vi "Cache_Hierarchy Global_Write.vi"(10 "Class Hierarchies":T1[](array[typedef]), 11 "Class Names":string[](array[string])) -> (3 "Hierarchy Map":map{string, string[]}(c390))   [LabVIEW 2019, in "ClassLoader.lvlib"]
uses:
  ClassLoader.lvlib
  Cache_Hierarchy Global.vi
  Ctl/Ctl_Hierarchy Cluster.ctl
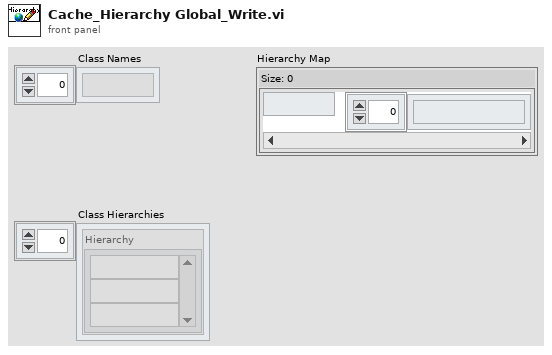
[diagram p1: front panel]
types:
  T1 = typedef "ClassLoader.lvlib/Ctl_Hierarchy Cluster.ctl" = cluster{"Hierarchy":string[]}
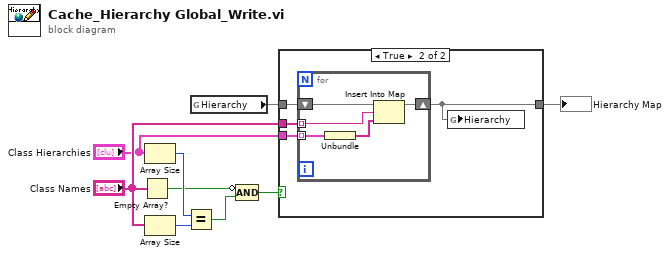
[diagram p0: block diagram]
diagram:
  n1 = Empty Array?(array="Class Names") -> (empty?=w2:bool)
  n2 = Array Size(array="Class Hierarchies") -> (size(s)=w4:i32)
  n3 = Array Size(array="Class Names") -> (size(s)=w5:i32)
  n4 = Equal?(x=w4, y=w5) -> (x = y?=w3:bool)
  n5 = global read "Cache_Hierarchy Global.vi" "Hierarchy"() -> (w9:map{string, string[]})
  n6 = Compound Arithmetic op=AND(invert w2, w3) -> (w1:bool)
  n7 = case shown="True" w1 {
    tunnel: "Class Names" -> [_ w14]
    tunnel: "Class Hierarchies" -> [_ w13]
    tunnel: w9 -> [w10 w12]
    tunnel: [w10 w11] -> w8
    frame False {
    }
    frame True {
      n8 = for {
        tunnel: w14 -> [w16] mode=indexing
        tunnel: w13 -> [w19] mode=indexing
        shift-right: [w17] -> w11
        shift-left: w12 -> [w18]
        n9 = Unbundle(w19) -> ("Hierarchy"=w15:string[])
        n10 = Insert Into Map(map in=w18, key=w16, value=w15) -> (map out=w17:map{string, string[]})  [unwired: 2 out]
      }
      n11 = global write "Cache_Hierarchy Global.vi" "Hierarchy"(w11) -> ()
    }
  }
  "Hierarchy Map" <- w8
